vi "Dashboard Main.vi"() -> ()   [LabVIEW 2012]
uses:
  <vilib>/Utility/config.llb/Read Key (String).vi
  <vilib>/Utility/config.llb/Read Key (I32).vi
  <vilib>/Utility/config.llb/Write Key (String).vi
  <vilib>/Utility/config.llb/Write Key (I32).vi
  <vilib>/Utility/inputDevices.llb/keyboardAcquire.vi
  <vilib>/Utility/config.llb/NI_LVConfig.lvlib
  <vilib>/Rock Robotics/WPI/Camera/WPI_CameraWhite Balance Values.ctl
panel:
  in  "Camera Settings":T1={"Frate Rate"=30, "Compression"=30, "Size"=1} {"Frate Rate" scale=1.0..30.0; "Size" items=["640x480", "320x240", "160x120"]}
  in  "Dashboard Tab":enum32{"Robot State"}(tab)
  out "Comp":bool
  out "Transfer":bool
  out "in flipper":bool
  out "middle":bool
  out "bottom":bool
  out "Robot IP":string
  out "Battery Value":dbl(slide) scale=0.0..14.0 scale format="%#_2e"
  out "Battery":sgl(graph)
  out "Frisbee Count":dbl
  out "zAvit":dbl(knob) scale=-20.0..50.0
  out "RPM":dbl(knob) scale=0.0..5000.0
  out "Cannon Angle":dbl
  out "Cannon RPM":dbl
  in  "Viewer":enum32{"Camera Image"}(tab)
  out "Mbps":dbl format="%#.1g"
  in  "Enable":bool
  in  "DB Camera Config":bool
  out "Mbps":bool
  out "fps":dbl format="%#.1g"
  out "Camera Image":T2(plugin-control)
  # "Robot IP:"
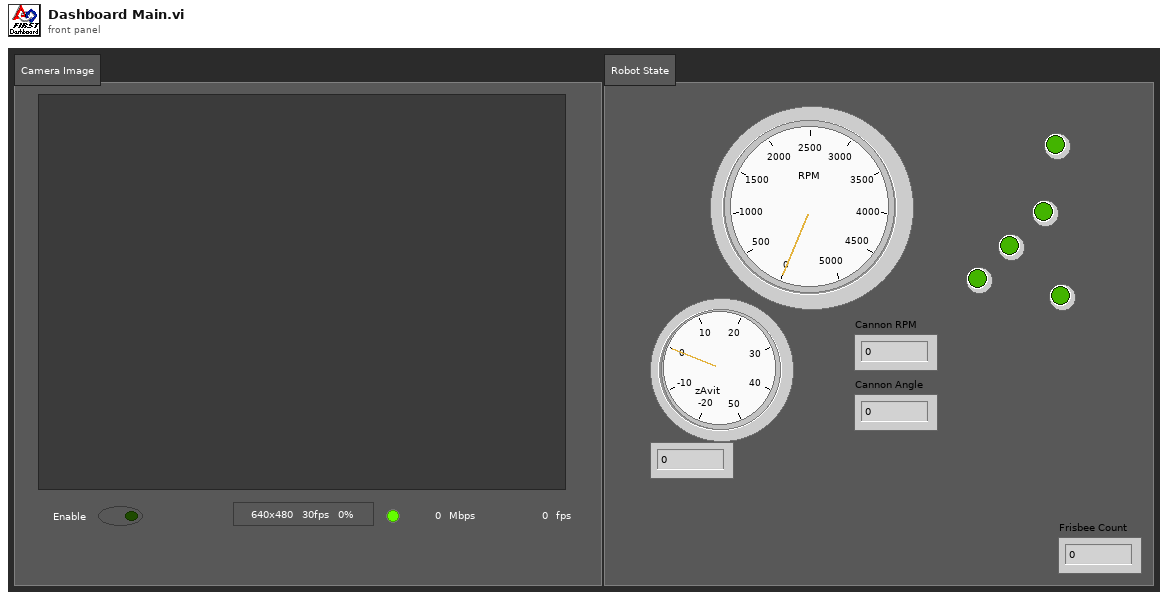
[diagram p1: front panel]
types:
  T1 = cluster{"Frate Rate":i32, "Compression":i32, "Size":u16}
  T2 = typedef "IMAQ Image.ctl" = refnum<image>
  T3 = typedef "Image Type" = u32
  T4 = typedef "WPI_CameraWhite Balance Values.ctl" = enum16{"Auto", "Fixed indoor", "Fixed outdoor 1", "Fixed outdoor 2", "Fixed fluorescent 1", "Fixed fluorescent 2", "Hold current"}
  T5 = typedef "WPI_CameraDevRef.ctl" = cluster{"Camera Address":string, "CameraStatus":errorcluster, "Acquire Image Notifier":refnum<notifier>}
  T6 = typedef "LVRectTypeDef.ctl" = cluster{"Left":i16, "Top":i16, "Right":i16, "Bottom":i16}
  T7 = cluster{"Competition mode":bool, "Robot Link":bool, "Autonomous":bool, "Enabled":bool, "E-Stop":bool, "Simulated":bool, "TestMode":bool, "Docked Window":bool}
  T8 = typedef "NI_LVConfig.lvlib/Config Data RefNum.ctl" = refnum<k1>
  T9 = enum16{"0", "1", "2", "3", "4", "5", "6", "7", "8", "9", "A", "B", "C", "D", "E", "F", "G", "H", "I", "J", "K", "L", "M", "N", "O", "P", "Q", "R", "S", "T", "U", "V", "W", "X", "Y", "Z", "F1", "F2", "F3", "F4", "F5", "F6", "F7", "F8", "F9", "F10", "F11", "F12", "F13", "F14", "F15", "ADD", "BACK", "BACKSLASH", "CAPITAL", "COMMA", "DECIMAL", "DELETE", "DIVIDE", "DOWN", "END", "EQUALS", "ESCAPE", "GRAVE (`)", "HOME", "INSERT", "LBRACKET", "LCONTROL", "LEFT", "L ALT", "LSHIFT", "LWIN", "MINUS", "MULTIPLY", "NEXT", "NUMLOCK", "NUMPAD_0", "NUMPAD_1", "NUMPAD_2", "NUMPAD_3", "NUMPAD_4", "NUMPAD_5", "NUMPAD_6", "NUMPAD_7", "NUMPAD_8", "NUMPAD_9", "PAUSE", "PERIOD", "PRIOR (PG UP)", "RBRACKET", "RCONTROL", "RETURN", "RIGHT", "R ALT", "RSHIFT", "RWIN", "SCROLL", "SEMICOLON", "SLASH", "SPACE", "SUBTRACT", "TAB", "UP", "ENTER (num pad)", "' (quote)"}
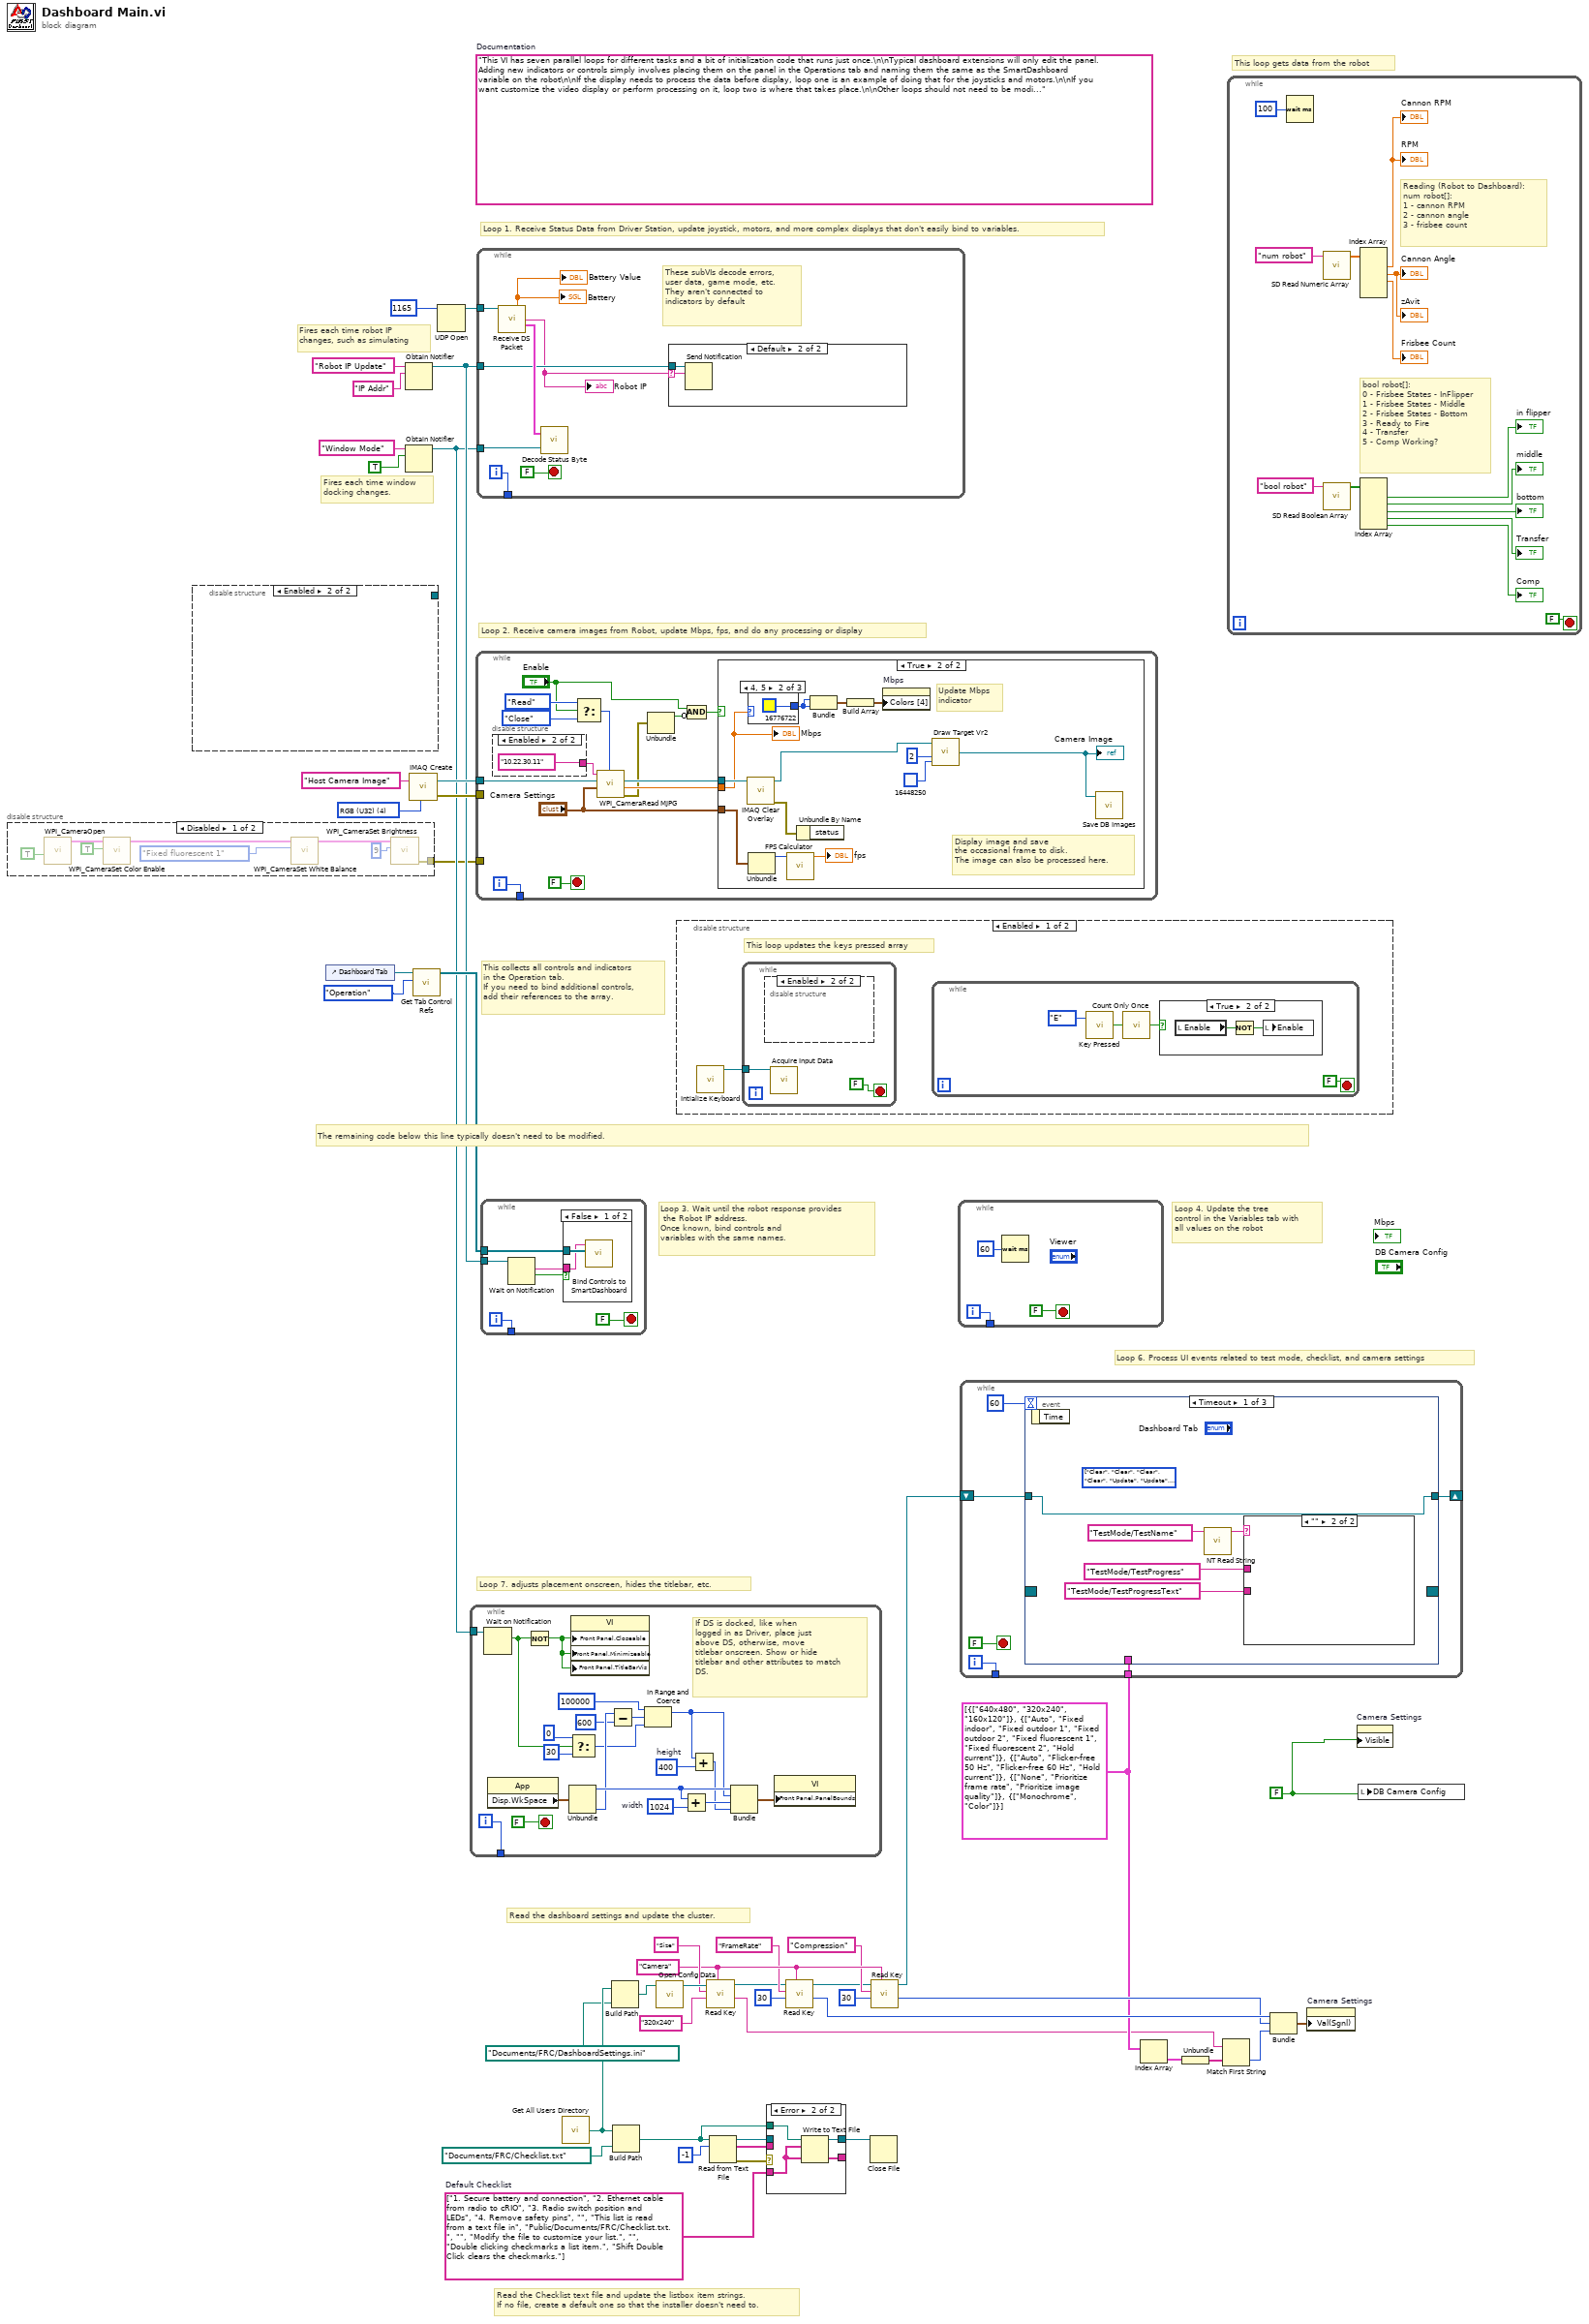
[diagram p0: block diagram]
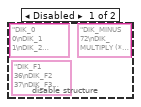
[diagram p3: hidden frame]
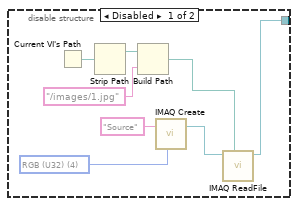
[diagram p6: hidden frame]
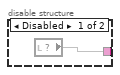
[diagram p8: hidden frame]
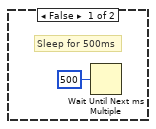
[diagram p9: hidden frame]
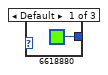
[diagram p10: hidden frame]
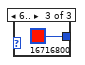
[diagram p11: hidden frame]
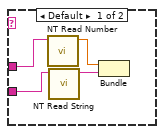
[diagram p13: hidden frame]
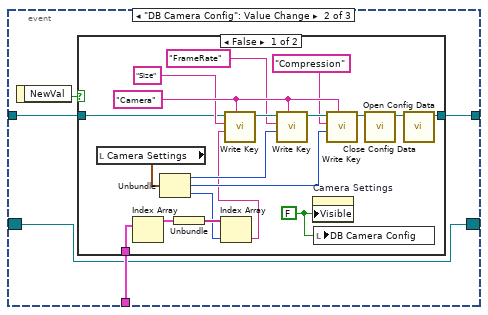
[diagram p14: hidden frame]
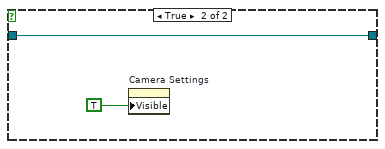
[diagram p15: hidden frame]
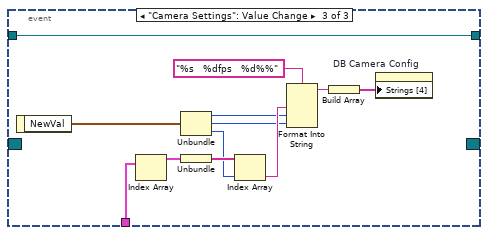
[diagram p16: hidden frame]
diagram:
  w20 = "Camera"
  w12 = cluster{string[]}[] [{["640x480", "320x240", "160x120"]}, {["Auto", "Fixed indoor", "Fixed outdoor 1", "Fixed outdoor 2", "Fixed fluorescent 1", "Fixed fluorescent 2", "Hold current"]}, {["Auto", "Flicker-free 50 Hz", "Flicker-free 60 Hz", "Hold current"]}, {["None", "Prioritize frame rate", "Prioritize image quality"]}, {["Monochrome", "Color"]}]
  w27 = string[] ["1. Secure battery and connection", "2. Ethernet cable from radio to cRIO", "3. Radio switch position and LEDs", "4. Remove safety pins", "", "This list is read from a text file in", "Public/Documents/FRC/Checklist.txt.", "", "Modify the file to customize your list.", "", "Double clicking checkmarks a list item.", "Shift Double Click clears the checkmarks."]  # Default Checklist
  w26 = FALSE ("Visible")
  (unwired) "This VI has seven parallel loops for different tasks and a bit of initialization code that runs just once.\n\nTypical dashboard extensions will only edit the panel. Adding new indicators or controls simply involves placing them on the panel in the Operations tab and naming them the same as the SmartDashboard variable on the robot\n\nIf the display needs to process the data before display, loop one is an example of doing that for the joysticks and motors.\n\nIf you want customize the video display or perform processing on it, loop two is where that takes place.\n\nOther loops should not need to be modified. They are pretty standard, and document the task they perform."  # Documentation
  w45 = T3 4 items=["Grayscale (U8)", "Grayscale (I16)", "Grayscale (SGL)", "Complex (CSG)", "RGB (U32)", "HSL (U32)", "RGB (U64)"] ("Image Type")
  # "This loop gets data from the robot"
  # "Fires each time robot IP\nchanges, such as simulating"
  # "Fires each time window\ndocking changes."
  # "Read the Checklist text file and update the listbox item strings.\nIf no file, create a default one so that the installer doesn't need to."
  # "This collects all controls and indicators\nin the Operation tab.\nIf you need to bind additional controls,\nadd their references to the array."
  # "The remaining code below this line typically doesn't need to be modified."
  # "Loop 6. Process UI events related to test mode, checklist, and camera settings"
  # "Read the dashboard settings and update the cluster."
  # "Loop 4. Update the tree\ncontrol in the Variables tab with\nall values on the robot"
  # "Loop 3. Wait until the robot response provides\n the Robot IP address.\nOnce known, bind controls and\nvariables with the same names."
  # "Loop 7. adjusts placement onscreen, hides the titlebar, etc."
  # "Loop 1. Receive Status Data from Driver Station, update joystick, motors, and more complex displays that don't easily bind to variables."
  # "Loop 2. Receive camera images from Robot, update Mbps, fps, and do any processing or display"
  n1 = disable-structure shown="Disabled" {
    disable-tunnel: [w48 _] -> w1
    frame Disabled {
      n2 = call <vilib>:"WPI_CameraOpen.vi"("Disallow Simulation"=TRUE) -> ("CameraDevRef"=w49:T5)  [unwired: 9 in, 1 out]
      n3 = call <vilib>:"WPI_CameraSet Color Enable.vi"("Color Enabled"=TRUE, "CameraDevRef"=w49) -> ("CameraDevRef Out"=w51:T5)  [unwired: 8 in, 1 out]
      n4 = call <vilib>:"WPI_CameraSet White Balance.vi"("White Balance"=WPI_CameraWhite_Balance_Values."Fixed fluorescent 1", "CameraDevRef"=w51) -> ("CameraDevRef Out"=w53:T5)  [unwired: 8 in, 1 out]
      n5 = call <vilib>:"WPI_CameraSet Brightness.vi"("Brightness"=9, "CameraDevRef"=w53) -> ("error out"=w48:errorcluster)  [unwired: 8 in, 1 out]
    }
    frame Enabled {
    }
  }
  n6 = disable-structure shown="Enabled" {
    disable-tunnel: [w60 _] -> _
    frame Disabled {
      w63 = T3 4 items=["Grayscale (U8)", "Grayscale (I16)", "Grayscale (SGL)", "Complex (CSG)", "RGB (U32)", "HSL (U32)", "RGB (U64)", "Grayscale (U16)"] ("Image Type")
      n7 = Current VI's Path() -> (path=w59:path)
      n8 = Strip Path(path=w59) -> (stripped path=w58:path)  [unwired: 1 out]
      n9 = Build Path(base path=w58, name or relative path="/images/1.jpg") -> (appended path=w56:path)
      n10 = call "IMAQ Create"("Image Name"="Source", "Image Type"=w63) -> ("New Image"=w62:T2)  [unwired: 2 in, 2 out]
      n11 = call "IMAQ ReadFile"("File Path"=w56, "Image"=w62) -> ("Image Out"=w60:T2)  [unwired: 5 in, 4 out]
    }
    frame Enabled {
    }
  }
  n12 = control-ref of="Dashboard Tab"() -> (w40:refnum<vi>)
  n13 = Obtain Notifier(name (unnamed)="Robot IP Update", notification data type="IP Addr" ("name (unnamed)")) -> (notifier out=w37:refnum<notifier>)  [unwired: 2 in, 2 out]
  n14 = Obtain Notifier(name (unnamed)="Window Mode", notification data type=TRUE) -> (notifier out=w31:refnum<notifier>)  [unwired: 2 in, 2 out]
  n15 = call "IMAQ Create"("Image Name"="Host Camera Image", "Image Type"=w45) -> ("New Image"=w43:T2, "error out"=w42:errorcluster)  [unwired: 2 in, 1 out]
  n16 = call <vilib>:"Get Tab Control Refs.vi"("Page Index"=enum32{"Operation", "Test"}."Operation" ("Dashboard Tab"), "TabControl in"=w40) -> ("ControlsOnPage"=w41:refnum<vi>[])  [unwired: 9 in]
  n17 = UDP Open(11:u16 1165 ("port")) -> (port=w46:refnum<k16>)  [unwired: 2 in, 4 out]
  n18 = while {
    tunnel: w31 -> [w82]
    tunnel: [w80] -> _
    i -> [w80]
    stop <- FALSE stop-if-true
    w73 = 1024  # width
    w76 = 400  # height
    # "If DS is docked, like when\nlogged in as Driver, place just\nabove DS, otherwise, move\ntitlebar onscreen. Show or hide\ntitlebar and other attributes to match\nDS."
    n19 = Wait on Notification(notifier=w82) -> (notification=w68:bool)  [unwired: 3 in, 3 out]
    n20 = property class="App"() -> ("Disp.WkSpace"=w79:T6)  [unwired: 2 in, 2 out]
    n21 = Not(x=w68) -> (.not. x?=w81:bool)
    n22 = Unbundle(w79) -> ("Left"=w77:i16, "Bottom"=w74:i16)  [unwired: 2 out]
    n23 = Select(t=0, s=w68, f=30) -> (s? t:f=w67:i32)
    n24 = property class="VI"("Front Panel.Closeable"=w81, "Front Panel.Minimizeable"=w81, "Front Panel.TitleBarVis"=w81) -> ()  [unwired: 2 in, 2 out]
    n25 = Subtract(x=w74, y=600) -> (x-y=w71:i32)
    n26 = In Range and Coerce(upper limit=100000, x=w71, lower limit=w67) -> (coerced(x)=w65:i32)  [unwired: 1 out]
    n27 = Add(x=w77, y=w73) -> (x+y=w78:i32)
    n28 = Add(x=w65, y=w76) -> (x+y=w75:i32)
    n29 = Bundle("Left"=w77, w65, w78, w75) -> (w64:cluster{"Left":i16, i32, i32, i32})  [unwired: 1 out]
    n30 = property class="VI"("Front Panel.PanelBounds"=w64) -> ()  [unwired: 2 in, 2 out]
  }
  n31 = while {
    tunnel: w43 -> [w93]
    tunnel: w42 -> [_]
    tunnel: [w96] -> _
    tunnel: w1 -> [_]
    i -> [w96]
    stop <- FALSE stop-if-true
    n32 = disable-structure shown="Enabled" {
      disable-tunnel: [w98 "10.22.30.11" ("address")] -> w95
      frame Disabled {
        n33 = local read item#-1() -> (w98)
      }
      frame Enabled {
      }
    }
    n34 = Select(t=enum16{"Read", "Reopen", "Close"}."Read" ("Operation"), s="Enable", f=enum16{"Read", "Reopen", "Close"}."Close" ("Operation")) -> (s? t:f=w88:enum16{"Read", "Reopen", "Close"})
    n35 = call <vilib>:"WPI_CameraRead MJPG.vi"("Operation"=w88, "Camera Settings"="Camera Settings", "Image"=w93, "address"=w95) -> ("error out"=w87:errorcluster, "Bandwidth (kbps)"=w91:dbl, "Image Out"=w92:T2)  [unwired: 5 in]
    n36 = Unbundle(w87) -> ("status"=w85:bool)  [unwired: 2 out]
    n37 = Compound Arithmetic op=AND("Enable", invert w85) -> (w84:bool)
    n38 = case shown="True" w84 {
      tunnel: "Camera Settings" -> [_ w106]
      tunnel: w92 -> [_ w109]
      tunnel: w91 -> [_ w108]
      frame False {
        # "Sleep for 500ms"
        n39 = Wait Until Next ms Multiple(millisecond multiple=u32 500) -> ()  [unwired: 1 out]
      }
      frame True {
        # "Display image and save\nthe occasional frame to disk.\nThe image can also be processed here."
        # "Update Mbps\nindicator"
        n40 = call "IMAQ Clear Overlay"("Image"=w109) -> ("error out"=w113:errorcluster, "Image Out"=w101:T2)  [unwired: 2 in, 7 out]
        n41 = case shown="4, 5" w108 {
          tunnel: [u32 6618880 ("Color Box") u32 16776722 ("Color Box") u32 16716800 ("Color Box")] -> w110
          frame Default {
          }
          frame 4, 5 {
          }
          frame 6.. {
          }
        }
        n42 = Unbundle(w106) -> ("Frate Rate"=w105:i32)  [unwired: 2 out]
        n43 = call "FPS Calculator.vi"("Average Count"=w105) -> ("fps"=→"fps":dbl)  [unwired: 10 in]
        n44 = Unbundle By Name(w113) -> ()  [unwired: 1 out]
        n45 = Bundle("Color Box"=w110, "Color Box"=w110) -> (w112:cluster{"Color Box":u32, "Color Box":u32})  [unwired: 1 out]
        n46 = Build Array(w112) -> (w111:cluster{"Color Box":u32, "Color Box":u32}[])
        n47 = property on="Mbps" class="Bool (strict)"("Colors [4]"=w111) -> ()  [unwired: 2 in, 2 out]
        n48 = call "Draw Target Vr2.vi"("Color"=u32 16448250, "Thickness"=2, "Original Image"=w101) -> ("Image Out"=w103:T2)
        "Camera Image" <- w103
        n49 = call "Save DB Images.vi"("Image"=w103) -> ()  [unwired: 2 in, 1 out]
        "Mbps" <- w108
      }
    }
  }
  n50 = while {
    tunnel: w46 -> [w122]
    tunnel: w37 -> [w118]
    tunnel: w31 -> [w120]
    tunnel: [w119] -> _
    i -> [w119]
    stop <- FALSE stop-if-true
    # "These subVIs decode errors, user data, game mode, etc.\nThey aren't connected to indicators by default"
    n51 = call "Receive DS Packet.vi"("Recv Socket"=w122) -> ("Battery"=→"Battery" →"Battery Value":sgl, "Robot IP Address"=w117:string, "Status"=w123:T7)  [unwired: 1 in, 11 out]
    "Robot IP" <- w117
    n52 = call "Decode Status Byte.vi"("Window Mode Notifier"=w120, "Status"=w123) -> ()  [unwired: 2 out]
    n53 = case shown="Default" w117 {
      selector: w117 -> [_ w125]
      tunnel: w118 -> [_ w126]
      frame "0.0.0.0" {
        # "Robot not responding, don't poll the variables"
      }
      frame Default {
        n54 = Send Notification(notification=w125, notifier=w126) -> ()  [unwired: 1 in, 2 out]
      }
    }
  }
  n55 = while {
    tunnel: w41 -> [w132]
    tunnel: w37 -> [w129]
    tunnel: [w127] -> _
    i -> [w127]
    stop <- FALSE stop-if-true
    n56 = Wait on Notification(notifier=w129) -> (notification=w128:string, timed out?=w130:bool)  [unwired: 3 in, 2 out]
    n57 = case shown="False" w130 {
      tunnel: w132 -> [w134 _]
      tunnel: w128 -> [w133 _]
      frame False {
        n58 = call <vilib>:"Bind Controls to SmartDashboard.vi"("Bound Control Refs"=w134, "Server IP Address"=w133) -> ()  [unwired: 10 in]
      }
      frame True {
      }
    }
  }
  n59 = call "Get All Users Directory.vi"() -> ("All User Path"=w25:path)
  n60 = Build Path(base path=w25, name or relative path=path "Documents/FRC/DashboardSettings.ini") -> (appended path=w24:path)
  n61 = Build Path(base path=w25, name or relative path=path "Documents/FRC/Checklist.txt") -> (appended path=w28:path)
  n62 = call <vilib>:"Open Config Data.vi"("configuration file path"=w24) -> ("refnum"=w23:T8)  [unwired: 8 in, 2 out]
  n63 = disable-structure shown="Enabled" {
    frame Enabled {
      # "This loop updates the keys pressed array"
      n64 = call <vilib>:"Intialize Keyboard.vi"() -> ("device ID"=w135:refnum<k1>)  [unwired: 10 in, 1 out]
      n65 = while {
        tunnel: w135 -> [w143]
        stop <- FALSE stop-if-true
        n66 = disable-structure shown="Enabled" {
          frame Disabled {
            (unwired) "DIK_MINUS                       72\nDIK_MULTIPLY (*)             73\nDIK_NEXT                          74\nDIK_NUMLOCK                  75\nDIK_NUMPAD0                  76\nDIK_NUMPAD1                  77\nDIK_NUMPAD2                  78\nDIK_NUMPAD3                  79\nDIK_NUMPAD4                  80\nDIK_NUMPAD5                  81\nDIK_NUMPAD6                  82\nDIK_NUMPAD7                  83\nDIK_NUMPAD8                  84\nDIK_NUMPAD9                  85\nDIK_PAUSE                       86\nDIK_PERIOD                     87\nDIK_PRIOR (pg up)           88\nDIK_RBRACKET ( ] )          89\nDIK_RCONTROL               90\nDIK_RETURN                    91\nDIK_RIGHT                       92\nDIK_RMENU (R ALT)         93\nDIK_RSHIFT (R shift)       94\nDIK_RWIN (R win)            95\nDIK_SCROLL                     96\nDIK_SEMICOLON              97\nDIK_SLASH                       98\nDIK_SPACE                       99\nDIK_SUBTRACT               100\nDIK_TAB                          101\nDIK_UP                            102\nDIR_ENTER(NUM)           103\nDIR_APOSTROPHY         104"
            (unwired) "DIK_F1                          36\nDIK_F2                          37\nDIK_F3                          38\nDIK_F4                          39\nDIK_F5                          40\nDIK_F6                          41\nDIK_F7                          42\nDIK_F8                          43\nDIK_F9                          44 \nDIK_F10                        45\nDIK_F11                        46\nDIK_F12                        47\nDIK_F13                        48 \nDIK_F14                        49\nDIK_F15                        50\nDIK_ADD                       51\nDIK_BACK                     52\nDIK_BACKSLASH           53\nDIK_CAPITAL                54\nDIK_COMMA                 55\nDIK_DECIMAL               56\nDIK_DELETE                  57\nDIK_DIVIDE                  58\nDIK_DOWN                   59\nDIK_END                       60\nDIK_EQUALS                 61\nDIK_ESCAPE                 62\nDIK_GRAVE (`)             63\nDIK_HOME                    64\nDIK_INSERT                  65\nDIK_LBRACKET             66\nDIK_LCONTROL            67\nDIK_LEFT                      68\nDIK_LMENU (L ALT)      69\nDIK_LSHIFT                  70\nDIK_LWIN                    71\n\n\n\n\n\n\n"
            (unwired) "DIK_0              0\nDIK_1              1\nDIK_2              2\nDIK_3              3\nDIK_4              4\nDIK_5              5\nDIK_6              6\nDIK_7              7\nDIK_8              8\nDIK_9              9\nDIK_A            10\nDIK_B             11\nDIK_C            12\nDIK_D            13\nDIK_E             14\nDIK_F             15\nDIK_G            16\nDIK_H            17\nDIK_I             18\nDIK_J             19\nDIK_K             20\nDIK_L             21\nDIK_M            22\nDIK_N            23\nDIK_O            24\nDIK_P             25\nDIK_Q            26\nDIK_R            27\nDIK_S             28\nDIK_T             29\nDIK_U            30\nDIK_V             31\nDIK_W           32\nDIK_X             33\nDIK_Y             34\nDIK_Z             35\n\n"
          }
          frame Enabled {
          }
        }
        n67 = call-poly <vilib>:"Acquire Input Data.vi"("device ID"=w143) -> ()  [unwired: 2 in, 17 out]
      }
      n68 = while {
        stop <- FALSE stop-if-true
        n69 = call "Key Pressed.vi"("key to be pressed"=T9."E") -> ("Was this key pressed"=w137:bool)  [unwired: 1 in]
        n70 = call "Count Only Once.vi"("InValue"=w137) -> ("Result"=w136:bool)
        n71 = case shown="True" w136 {
          frame False {
          }
          frame True {
            n72 = local read "Enable"() -> (w141:bool)
            n73 = Not(x=w141) -> (.not. x?=w140:bool)
            n74 = local write "Enable"(w140) -> ()
          }
        }
      }
    }
    frame Disabled {
    }
  }
  n75 = call-poly <vilib>:"Read Key.vi"("section"=w20, "default value"="320x240", "key"="Size", "refnum"=w23) -> ("value"=w10:string, "refnum out"=w5:T8)  [unwired: 2 in, 4 out]
  n76 = Read from Text File(file (use dialog)=w28, count=-1 ("timeout ms (25000)")) -> (refnum out=w7:refnum<file>, text=w29:string[], error out=w30:errorcluster)  [unwired: 2 in, 1 out]
  n77 = case shown="Error" w30 {
    tunnel: w29 -> [w145 _]
    tunnel: [w145 w147] -> _
    tunnel: w27 -> [_ w147]
    tunnel: w28 -> [_ w148]
    tunnel: [w144 w146] -> w6
    tunnel: w7 -> [w144 _]
    frame No Error {
    }
    frame Error {
      n78 = Write to Text File(file (use dialog)=w148, text=w147) -> (refnum out=w146:refnum<file>)  [unwired: 2 in, 2 out]
    }
  }
  n79 = call-poly <vilib>:"Read Key.vi"("section"=w20, "default value"=30, "key"="FrameRate", "refnum"=w5) -> ("value"=w15:i32, "refnum out"=w4:T8)  [unwired: 1 in, 5 out]
  n80 = Close File(refnum=w6) -> ()  [unwired: 1 in, 2 out]
  n81 = call-poly <vilib>:"Read Key.vi"("section"=w20, "default value"=30, "key"="Compression", "refnum"=w4) -> ("value"=w14:i32, "refnum out"=w2:T8)  [unwired: 1 in, 5 out]
  n82 = while {
    tunnel: [w149] -> _
    i -> [w149]
    stop <- FALSE stop-if-true
    n83 = Wait (ms)(milliseconds to wait=u32 60) -> ()  [unwired: 1 out]
  }
  n84 = while {
    tunnel: w12 -> [w155]
    shift-right: [w154] -> _
    shift-left: w2 -> [w153]
    tunnel: [w152] -> _
    i -> [w152]
    stop <- FALSE stop-if-true
    n85 = event shown="[0] Timeout" {
      selector: _ -> [_ w167 _]
      dyn-events: [_ w167 _] -> _
      timeout: u32 60 ("milliseconds to wait") -> [_ _ _]
      tunnel: w155 -> [_ w170 w200]
      tunnel: [w158 w169 w193] -> w154
      tunnel: w153 -> [w158 w168 w193]
      event Timeout {
        (unwired) enum16{"Update", "Clear"}[] [enum."Clear", enum."Clear", enum."Clear", enum."Clear", enum."Update", enum."Update", enum."Clear"] items=["Update", "Clear"]
        n86 = event-data() -> ()  [unwired: 1 in, 1 out]
        n87 = call <vilib>:"NT Read String.vi"("Name"="TestMode/TestName") -> ("String"=w161:string)  [unwired: 9 in, 1 out]
        n88 = case shown="\"\"" w161 {
          tunnel: "TestMode/TestProgress" ("Name") -> [w164 _]
          tunnel: "TestMode/TestProgressText" ("Name") -> [w163 _]
          frame Default {
            n89 = call <vilib>:"NT Read Number.vi"("Name"=w164) -> ("Numeric"=w165:dbl)  [unwired: 9 in, 1 out]
            n90 = call <vilib>:"NT Read String.vi"("Name"=w163) -> ("String"=w166:string)  [unwired: 9 in, 1 out]
            n91 = Bundle("Numeric"=w165, "String"=w166) -> ()  [unwired: 1 in, 1 out]
          }
          frame "" {
          }
        }
      }
      event "DB Camera Config": Value Change {
        n92 = event-data() -> ("NewVal"=w171:bool)  [unwired: 1 in]
        n93 = case shown="False" w171 {
          tunnel: w170 -> [w180 _]
          tunnel: [w173 w191] -> w169
          tunnel: w168 -> [w172 w191]
          frame False {
            w187 = "Camera"
            w190 = FALSE ("Visible")
            n94 = local read "Camera Settings"() -> (w179:T1)
            n95 = Index Array(array=w180) -> (element=w183:cluster{string[]})  [unwired: 1 in]
            n96 = Unbundle(w179) -> ("Frate Rate"=w178:i32, "Compression"=w177:i32, "Size"=w181:u16)
            n97 = Unbundle(w183) -> (w182:string[])
            n98 = Index Array(array=w182, index=w181) -> (element=w176:string)
            n99 = call-poly <vilib>:"Write Key.vi"("section"=w187, "value"=w176, "key"="Size", "refnum"=w172) -> ("refnum out"=w189:T8)  [unwired: 2 in, 5 out]
            n100 = call-poly <vilib>:"Write Key.vi"("section"=w187, "value"=w178, "key"="FrameRate", "refnum"=w189) -> ("refnum out"=w188:T8)  [unwired: 1 in, 6 out]
            n101 = property on="Camera Settings" class="Clust (strict)"("Visible"=w190) -> ()  [unwired: 2 in, 2 out]
            n102 = local write "DB Camera Config"(w190) -> ()
            n103 = call-poly <vilib>:"Write Key.vi"("section"=w187, "value"=w177, "key"="Compression", "refnum"=w188) -> ("refnum out"=w174:T8)  [unwired: 1 in, 6 out]
            n104 = call <vilib>:"Close Config Data.vi"("refnum"=w174) -> ("file path"=w175:path)  [unwired: 2 in, 8 out]
            n105 = call <vilib>:"Open Config Data.vi"("configuration file path"=w175) -> ("refnum"=w173:T8)  [unwired: 8 in, 2 out]
          }
          frame True {
            n106 = property on="Camera Settings" class="Clust (strict)"("Visible"=TRUE) -> ()  [unwired: 2 in, 2 out]
          }
        }
      }
      event "Camera Settings": Value Change {
        n107 = event-data() -> ("NewVal"=w204:T1)  [unwired: 1 in]
        n108 = Index Array(array=w200) -> (element=w199:cluster{string[]})  [unwired: 1 in]
        n109 = Unbundle(w204) -> ("Frate Rate"=w195:i32, "Compression"=w194:i32, "Size"=w197:u16)
        n110 = Unbundle(w199) -> (w198:string[])
        n111 = Index Array(array=w198, index=w197) -> (element=w196:string)
        n112 = Format Into String(format string="%s   %dfps   %d%%", w196, w195, w194) -> (resulting string=w201:string)  [unwired: 2 in, 1 out]
        n113 = Build Array(w201) -> (w202:string[])
        n114 = property on="DB Camera Config" class="Bool (strict)"("Strings [4]"=w202) -> ()  [unwired: 2 in, 2 out]
      }
    }
  }
  n115 = Index Array(array=w12) -> (element=w13:cluster{string[]})  [unwired: 1 in]
  n116 = Unbundle(w13) -> (w11:string[])
  n117 = Match First String(2:w11, 3:w10) -> (0:w9:i32)  [unwired: 1 out]
  n118 = while {
    stop <- FALSE stop-if-true
    # "bool robot[]:\n0 - Frisbee States - InFlipper\n1 - Frisbee States - Middle\n2 - Frisbee States - Bottom\n3 - Ready to Fire\n4 - Transfer\n5 - Comp Working?"
    # "Reading (Robot to Dashboard):\nnum robot[]:\n1 - cannon RPM\n2 - cannon angle\n3 - frisbee count"
    n119 = Wait (ms)(milliseconds to wait=u32 100) -> ()  [unwired: 1 out]
    n120 = call <vilib>:"SD Read Numeric Array.vi"("Name"="num robot") -> ("Numeric Array"=w214:dbl[])  [unwired: 8 in, 2 out]
    n121 = call <vilib>:"SD Read Boolean Array.vi"("Name"="bool robot") -> ("Boolean Array"=w215:bool[])  [unwired: 8 in, 2 out]
    n122 = Index Array(array=w214) -> (element #1=→"Cannon RPM" →"RPM":dbl, element #2=→"Cannon Angle" →"zAvit":dbl, element #3=→"Frisbee Count":dbl)  [unwired: 5 in, 2 out]
    n123 = Index Array(array=w215) -> (element #1=→"in flipper":bool, element #2=→"middle":bool, element #3=→"bottom":bool, element #4=→"Transfer":bool, element #5=→"Comp":bool)  [unwired: 5 in]
  }
  n124 = Bundle("value"=w15, "value"=w14, "index"=w9) -> (w3:cluster{"value":i32, "value":i32, "index":i32})  [unwired: 1 out]
  n125 = property on="Camera Settings" class="Clust (strict)"("Val(Sgnl)"=w3) -> ()  [unwired: 2 in, 2 out]
  n126 = property on="Camera Settings" class="Clust (strict)"("Visible"=w26) -> ()  [unwired: 2 in, 2 out]
  n127 = local write "DB Camera Config"(w26) -> ()
